vi "Manual heater.vi"() -> ()   [LabVIEW 2015]
panel:
  in  "Heater %":dbl
  in  "PID":cluster{"P":dbl, "I":dbl, "D":dbl}
  in  "Control":bool
  in  "Sensor":i32=1
  in  "VISA Resource Name":refnum<visa-resource-name>
  in  "Stop Button":bool
  out "Heater":dbl(graph)
  out "Temperaturte":dbl(graph)
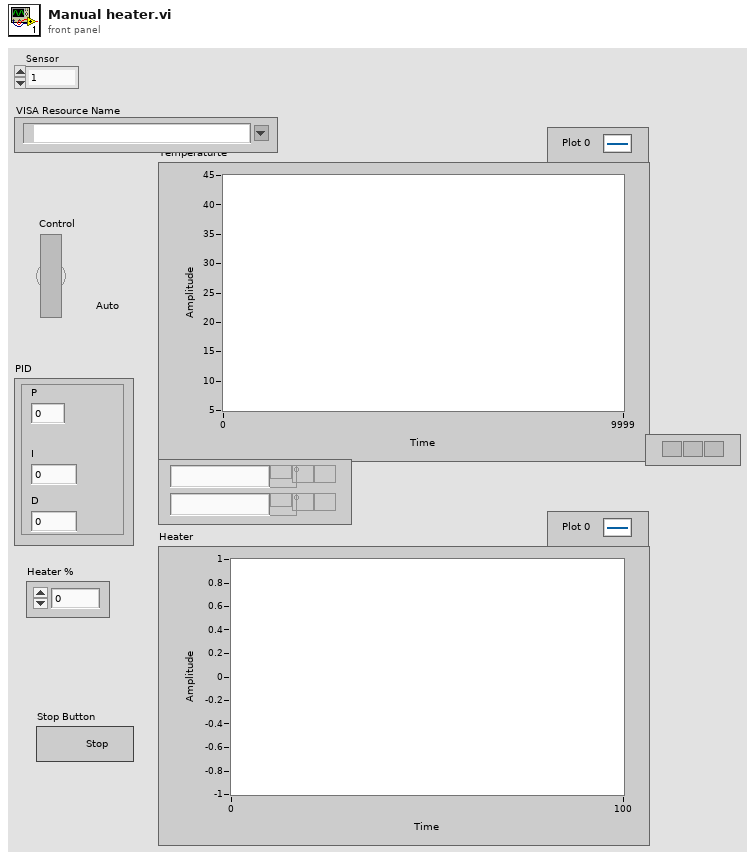
[diagram p1: front panel]
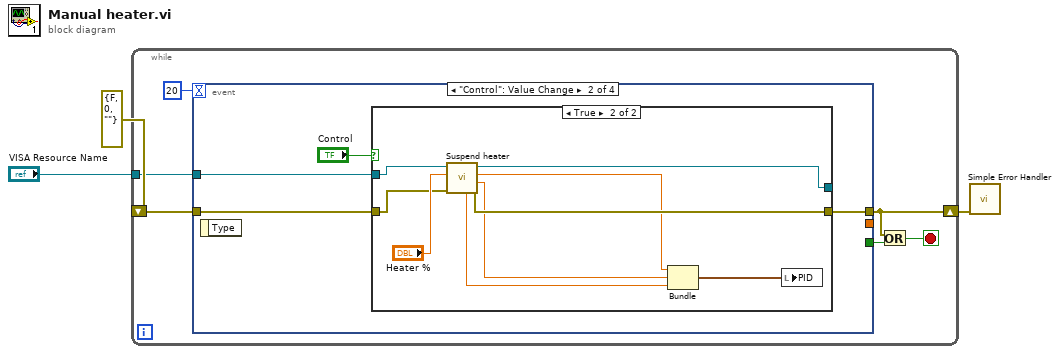
[diagram p0: block diagram]
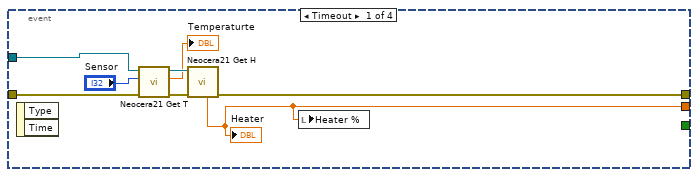
[diagram p2: hidden frame]
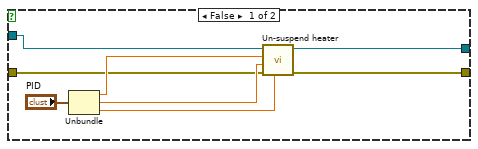
[diagram p3: hidden frame]
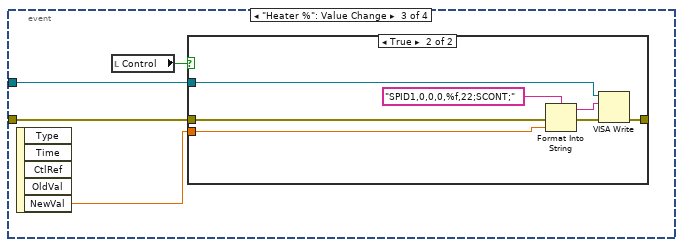
[diagram p4: hidden frame]
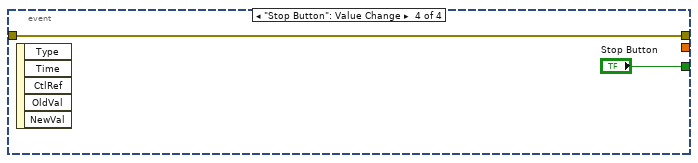
[diagram p6: hidden frame]
diagram:
  n1 = while {
    tunnel: "VISA Resource Name" -> [w8]
    shift-right: [w6] -> w2
    shift-left: errorcluster {"status"=FALSE, "code"=0, "source"=""} ("error out") -> [w7]
    stop <- w9 stop-if-true
    n2 = event shown="[1] \"Control\": Value Change" {
      selector: _ -> [_ _ _ _]
      dyn-events: _ -> [_ _ _ _]
      timeout: 20 -> [_ _ _ _]
      tunnel: w8 -> [w17 w18 w40 _]
      tunnel: w7 -> [w16 w20 w41 w51]
      tunnel: [w13 w19 _ w51] -> w6
      tunnel: [_ _ _ "Stop Button"] -> w5
      tunnel: [w10 _ _ _] -> _
      event Timeout {
        n3 = event-data() -> ()  [unwired: 1 in, 2 out]
        n4 = call "Neocera21 Get T.vi"("error in (no error)"=w16, "Sensor"="Sensor", "VISA Resource Name"=w17) -> ("error out"=w14:errorcluster, "Temperature"=→"Temperaturte":dbl, "VISA Resource Name Out"=w15:refnum<visa-resource-name>)  [unwired: 5 in, 1 out]
        n5 = call "Neocera21 Get H.vi"("error in (no error)"=w14, "VISA Resource Name"=w15) -> ("error out"=w13:errorcluster, "Heat %"=w10:dbl)  [unwired: 4 in, 4 out]
        "Heater" <- w10
        n6 = local write "Heater %"(w10) -> ()
      }
      event "Control": Value Change {
        n7 = event-data() -> ()  [unwired: 1 in, 1 out]
        n8 = case shown="True" "Control" {
          tunnel: w20 -> [w24 w31]
          tunnel: w18 -> [w23 w32]
          tunnel: [w29 w38] -> w19
          tunnel: [w28 w37] -> _
          frame False {
            n9 = Unbundle("PID") -> ("P"=w27:dbl, "I"=w26:dbl, "D"=w22:dbl)
            n10 = call "Un-suspend heater.vi"("D"=w22, "error in (no error)"=w24, "I"=w26, "P"=w27, "VISA Refnum in"=w23) -> ("error out"=w29:errorcluster, "VISA Refnum out"=w28:refnum<visa-resource-name>)  [unwired: 5 in]
          }
          frame True {
            n11 = call "Suspend heater.vi"("error in (no error)"=w31, "Heater %"="Heater %", "VISA resource name"=w32) -> ("error out"=w38:errorcluster, "I"=w34:dbl, "P"=w35:dbl, "VISA resource name out"=w37:refnum<visa-resource-name>, "D"=w30:dbl)  [unwired: 3 in, 1 out]
            n12 = Bundle("P"=w35, "I"=w34, "D"=w30) -> (w33:cluster{"P":dbl, "I":dbl, "D":dbl})  [unwired: 1 in]
            n13 = local write "PID"(w33) -> ()
          }
        }
      }
      event "Heater %": Value Change {
        n14 = event-data() -> ("NewVal"=w39:dbl)  [unwired: 1 in, 4 out]
        n15 = local read "Control"() -> (w42:bool)
        n16 = case shown="True" w42 {
          tunnel: w41 -> [w43 w45]
          tunnel: w40 -> [_ w44]
          tunnel: [w43 w48] -> _
          tunnel: w39 -> [_ w46]
          frame False {
          }
          frame True {
            n17 = Format Into String(format string="SPID1,0,0,0,%f,22;SCONT;", error in=w45, w46) -> (resulting string=w49:string, error out=w50:errorcluster)  [unwired: 1 in]
            n18 = VISA Write(VISA resource name=w44, write buffer=w49, error in (no error)=w50) -> (error out=w48:errorcluster)  [unwired: 2 out]
          }
        }
      }
      event "Stop Button": Value Change {
        n19 = event-data() -> ()  [unwired: 1 in, 5 out]
      }
    }
    n20 = Or(x=w6, y=w5) -> (x .or. y?=w9:bool)
  }
  n21 = call <vilib>:"Simple Error Handler.vi"("error in (no error)"=w2) -> ()  [unwired: 4 in, 5 out]
